vi "filter tags by type.vi"(10 "allowable types":T1[](array[typedef]), 11 "tags in":refnum<class "data bus tag description.lvclass">[](array[class])) -> (3 "filtered tags":refnum<class "data bus tag description.lvclass">[](array[class]))   [LabVIEW 2013, in "data bus tag description.lvclass"]
doc: "Filters a list of tags by type, eliminating all tags which do not match the desired set of types."
uses:
  data bus tag description.lvclass
  Data Type.ctl
  data bus tag description.lvclass/data bus tag description.ctl
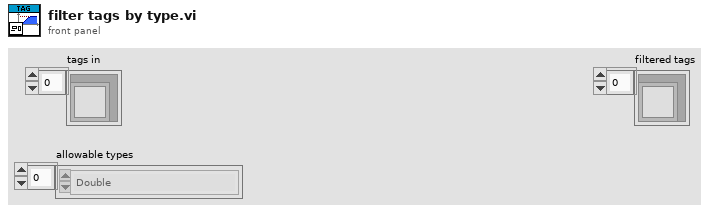
[diagram p1: front panel]
types:
  T1 = typedef "data bus tag description.lvclass/Data Type.ctl" = enum16{"Double", "I64", "Boolean", "Array of Double", "Array of I64", "Variant"}
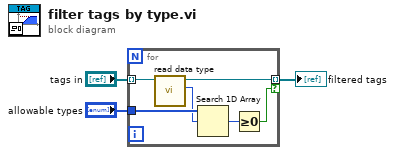
[diagram p0: block diagram]
diagram:
  n1 = for {
    tunnel: [w8] -> w3 mode=indexing if=w4
    tunnel: "tags in" -> [w9] mode=indexing
    tunnel: "allowable types" -> [w7]
    n2 = call "read data type.vi"("system tag in"=w9) -> ("data type"=w6:T1, "system tag out"=w8:refnum<class "data bus tag description.lvclass">)  [unwired: 8 in, 1 out]
    n3 = Search 1D Array(1D array=w7, element=w6) -> (index of element=w5:i32)  [unwired: 1 in]
    n4 = Greater Or Equal To 0?(x=w5) -> (x >= 0?=w4:bool)
  }
  "filtered tags" <- w3
